vi "Theremin Frequency.vi"(4 "Min Freq":dbl, 5 "Min Amp":dbl, 6 "Max Freq":dbl, 7 "Max Amp":dbl, 10 "Input Amp":dbl) -> (2 "Output Freq":dbl)   [LabVIEW 2012]
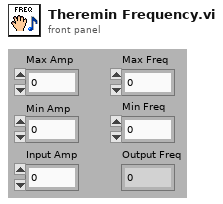
[diagram p1: front panel]
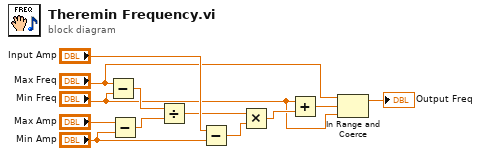
[diagram p0: block diagram]
diagram:
  n1 = Subtract(x="Max Freq", y="Min Freq") -> (x-y=w11:dbl)
  n2 = Subtract(x="Max Amp", y="Min Amp") -> (x-y=w10:dbl)
  n3 = Divide(x=w11, y=w10) -> (x/y=w7:dbl)
  n4 = Subtract(x="Input Amp", y="Min Amp") -> (x-y=w6:dbl)
  n5 = Multiply(x=w7, y=w6) -> (x*y=w5:dbl)
  n6 = Add(x="Min Freq", y=w5) -> (x+y=w4:dbl)
  n7 = In Range and Coerce(upper limit="Max Freq", x=w4, lower limit="Min Freq") -> (coerced(x)=→"Output Freq":dbl)  [unwired: 1 out]
